vi "Forward Dynamics.vi"(10 "Scale":dbl, 11 "Tension":dbl[](array[numeric])) -> (3 "Robot Force":dbl[](array[numeric]))   [LabVIEW 2021]
uses:
  <vilib>/Analysis/baseanly.llb/A x Vector.vi
  <vilib>/Analysis/Matrix/Numeric/Conversions/Array To Matrix - RA2.vi
  <vilib>/Analysis/Matrix/NI_Matrix.lvlib
  <vilib>/Analysis/NI_AALBase.lvlib
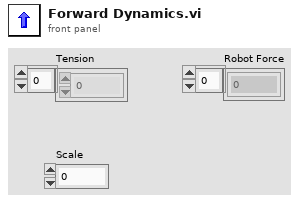
[diagram p1: front panel]
types:
  T1 = typedef "NI_Matrix.lvlib/RealMatrix.ctl" = dbl[][]
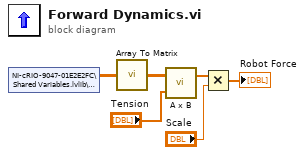
[diagram p0: block diagram]
diagram:
  n1 = shared-variable "NI-cRIO-9047-01E2E2FC\\Shared Variables.lvlib\\Jacobian"() -> (w3:dbl[][])  [unwired: 1 in, 1 out]
  n2 = call-poly <vilib>:"Array To Matrix.vi"("Real 2D Array"=w3) -> ("Real Matrix"=w4:T1)
  n3 = call-poly <vilib>:"A x B.vi"("Vector"="Tension", "A"=w4) -> ("A x Vector"=w5:dbl[])  [unwired: 1 out]
  n4 = Multiply ("Multiply.vi")(x=w5, y="Scale") -> (x*y=→"Robot Force":dbl[])
